vi "TDS DCPS Set Output State.vi"(8 "error in (no error)":errorcluster, 9 "Output State":bool, 10 "Signal InstConfig":string, 11 "Address":string) -> (0 "error out":errorcluster)   [LabVIEW 2025, in "Interface Functions.lvlib"]
uses:
  Interface Functions.lvlib
panel:
  # "DCPS Set Output State"
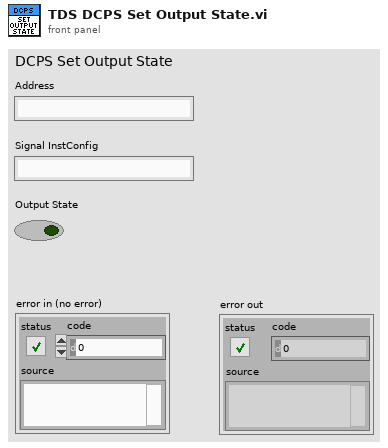
[diagram p1: front panel]
types:
  T1 = typedef "Control 1" = cluster{"Channel":i32, "Current Limit Mode":enum16{"REGULATE", "TRIP"}}
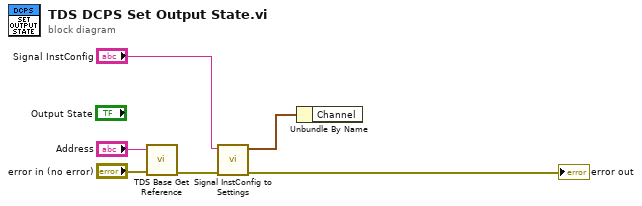
[diagram p0: block diagram]
diagram:
  n1 = call "TDS Base Get Reference.vi"("error in (no error)"="error in (no error)", "Address"="Address") -> ("error out"=w4:errorcluster)  [unwired: 8 in, 1 out]
  n2 = call "Signal InstConfig to Settings.vi"("error in (no error)"=w4, "Signal InstConfig"="Signal InstConfig") -> ("error out"=→"error out":errorcluster, "Settings"=w2:T1)  [unwired: 8 in]
  n3 = Unbundle By Name(w2) -> ()  [unwired: 1 out]
